vi "Initialize Attributes Core.vi"(8 "error in (no error)":errorcluster, 10 "Attribute Data":variant, 11 "BNT_ULx-MCSV in":refnum<class "BNT_ULx-MCSV.lvclass">) -> (0 "error out":errorcluster, 2 "MandatoryParameters":cluster{"Parameter":string, "found?":bool}[](array[cluster]), 3 "BNT_ULx-MCSV out":refnum<class "BNT_ULx-MCSV.lvclass">)   [LabVIEW 2021, in "BNT_ULx.lvlib" / "BNT_ULx-MCSV.lvclass"]
doc: "Initialize object attribute.\n\nUnique resources should be allocated elsewhere!"
uses:
  BNT_ULx-MCSV.lvclass
  C:/Users/Holger/Documents/LVP/CSPP/CSPP-Template/Packages/CSPP_Core/Actors/CSPP_DeviceActor/CSPP_DeviceActor.lvclass
  C:/Users/Holger/Documents/LVP/CSPP/CSPP-Template/Packages/CSPP_Core/Actors/CSPP_BaseActor/CSPP_BaseActor.lvclass
  CSPP_Core/Actors/CSPP_DeviceActor/CSPP_DeviceActor.lvclass/CSPP_DeviceActor.ctl
  CSPP_Core/Actors/CSPP_BaseActor/CSPP_BaseActor.lvclass/CSPP_BaseActor.ctl
  BNT_ULx-MCSV.lvclass/BNT_ULx-MCSV.ctl
  CSPP_Core/Libraries/Base/Severity.ctl
  CSPP_Core/Actors/CSPP_DeviceActor/CSPP_DeviceActor.lvclass
  CSPP_Core/Classes/CSPP_BaseClasses/Factory/CSPP_Factory.lvclass
  CSPP_Core/Actors/CSPP_BaseActor/CSPP_BaseActor.lvclass
  CSPP_Core/Libraries/Utilities/CSPP_Utilities.lvlib
  CSPP_Core/Libraries/Base/CSPP_Base.lvlib
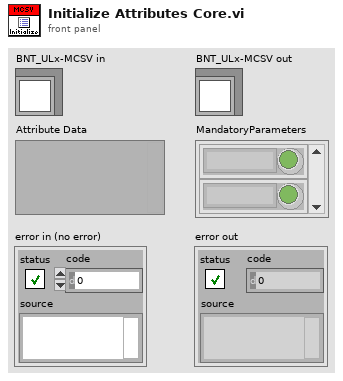
[diagram p1: front panel]
types:
  T1 = typedef "CSPP_Base.lvlib/Severity.ctl" = enum16{"emergency", "alert", "critical", "error", "warning", "notice", "info", "debug"}
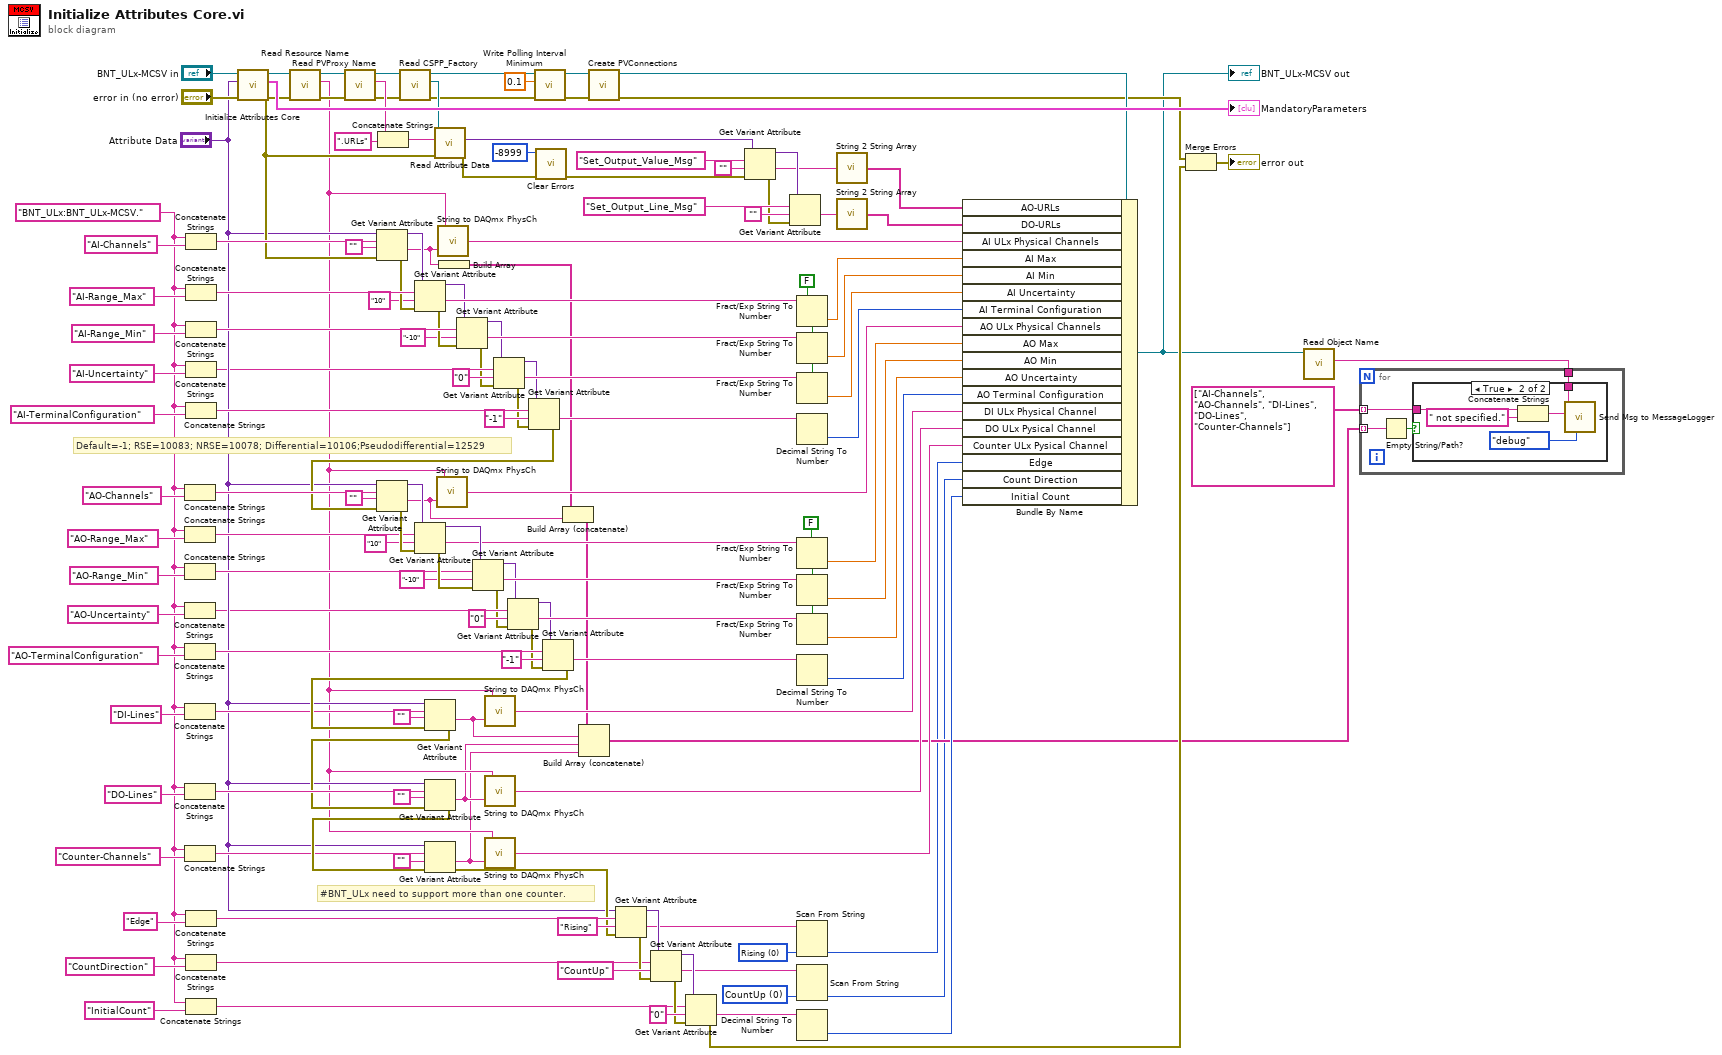
[diagram p0: block diagram]
diagram:
  w2 = 0 items=["CountUp", "CountDown"] ("Count Direction")
  w5 = 0 items=["Rising", "Falling"] ("Edge")
  w26 = FALSE ("use system decimal point (T)")
  w36 = FALSE ("use system decimal point (T)")
  w22 = "BNT_ULx:BNT_ULx-MCSV."
  # "#BNT_ULx need to support more than one counter."
  # "Default=-1; RSE=10083; NRSE=10078; Differential=10106;Pseudodifferential=12529"
  n1 = Concatenate Strings(w22, "AO-Channels" ("string")) -> (w130:string)
  n2 = Concatenate Strings(w22, "AO-Range_Max" ("string")) -> (w121:string)
  n3 = Concatenate Strings(w22, "AO-Range_Min" ("string")) -> (w124:string)
  n4 = Concatenate Strings(w22, "AO-Uncertainty" ("string")) -> (w28:string)
  n5 = Concatenate Strings(w22, "AO-TerminalConfiguration" ("string")) -> (w127:string)
  n6 = Concatenate Strings(w22, "DI-Lines" ("string")) -> (w108:string)
  n7 = Concatenate Strings(w22, "DO-Lines" ("string")) -> (w109:string)
  n8 = Concatenate Strings(w22, "Counter-Channels" ("string")) -> (w61:string)
  n9 = Concatenate Strings(w22, "AI-Channels" ("string")) -> (w138:string)
  n10 = Concatenate Strings(w22, "AI-Range_Max" ("string")) -> (w149:string)
  n11 = Concatenate Strings(w22, "AI-Range_Min" ("string")) -> (w146:string)
  n12 = Concatenate Strings(w22, "AI-Uncertainty" ("string")) -> (w38:string)
  n13 = Concatenate Strings(w22, "AI-TerminalConfiguration" ("string")) -> (w143:string)
  n14 = Concatenate Strings(w22, "Edge" ("string")) -> (w73:string)
  n15 = Concatenate Strings(w22, "CountDirection" ("string")) -> (w68:string)
  n16 = Concatenate Strings(w22, "InitialCount" ("string")) -> (w70:string)
  n17 = call-parent "Initialize Attributes Core.vi"("error in (no error)"="error in (no error)", "Attribute Data"="Attribute Data", "CSPP_DeviceActor in"="BNT_ULx-MCSV in") -> ("error out"=w54:errorcluster, "MandatoryParameters"=→"MandatoryParameters":cluster{"Parameter":string, "found?":bool}[], "CSPP_DeviceActor out"=w134:refnum<class "BNT_ULx-MCSV.lvclass">)  [unwired: 6 in]
  n18 = call "Read Resource Name.vi"("error in (no error)"=w54, "CSPP_DeviceActor in"=w134) -> ("error out"=w55:errorcluster, "Resource Name"=w18:string, "CSPP_DeviceActor out"=w106:refnum<class "BNT_ULx-MCSV.lvclass">)  [unwired: 7 in]
  n19 = call "Read PVProxy Name.vi"("error in (no error)"=w55, "CSPP_BaseActor in"=w106) -> ("error out"=w47:errorcluster, "PVProxy Name"=w101:string, "CSPP_BaseActor out"=w50:refnum<class "BNT_ULx-MCSV.lvclass">)  [unwired: 7 in]
  n20 = Get Variant Attribute(Variant="Attribute Data", name=w138, default value (empty Variant)="", error in=w54) -> (duplicate Variant=w137:variant, value=w14:string, error out=w136:errorcluster)  [unwired: 1 out]
  n21 = Concatenate Strings(w101, ".URLs" ("string")) -> (w103:string)
  n22 = call "Read CSPP_Factory.vi"("error in (no error)"=w47, "CSPP_BaseActor in"=w50) -> ("error out"=w46:errorcluster, "CSPP_Factory"=w48:refnum<class "CSPP_Factory.lvclass">, "CSPP_BaseActor out"=w49:refnum<class "BNT_ULx-MCSV.lvclass">)  [unwired: 7 in]
  n23 = Get Variant Attribute(Variant=w137, name=w149, default value (empty Variant)="10" ("string"), error in=w136) -> (duplicate Variant=w147:variant, value=w148:string, error out=w145:errorcluster)  [unwired: 1 out]
  n24 = call-dynamic "Read Attribute Data.vi"("error in (no error)"=w54, "Object Name"=w103, "CSPP_Factory in"=w48) -> ("error out"=w105:errorcluster, "Attribute Data"=w99:variant)  [unwired: 6 in, 1 out]
  n25 = call "String to DAQmx PhysCh.vi"("Channel String"=w14, "Resource Name"=w18) -> ("DAQmx Physical Channels"=w19:string)
  n26 = Build Array(w14) -> (w12:string[])
  n27 = Get Variant Attribute(Variant=w147, name=w146, default value (empty Variant)="-10" ("string"), error in=w145) -> (duplicate Variant=w33:variant, value=w144:string, error out=w32:errorcluster)  [unwired: 1 out]
  n28 = Get Variant Attribute(Variant=w33, name=w38, default value (empty Variant)="0" ("string"), error in=w32) -> (duplicate Variant=w35:variant, value=w39:string, error out=w34:errorcluster)  [unwired: 1 out]
  n29 = Get Variant Attribute(Variant=w35, name=w143, default value (empty Variant)="-1" ("string"), error in=w34) -> (value=w142:string, error out=w116:errorcluster)  [unwired: 2 out]
  n30 = Get Variant Attribute(Variant="Attribute Data", name=w130, default value (empty Variant)="", error in=w116) -> (duplicate Variant=w131:variant, value=w13:string, error out=w132:errorcluster)  [unwired: 1 out]
  n31 = Get Variant Attribute(Variant=w131, name=w121, default value (empty Variant)="10" ("string"), error in=w132) -> (duplicate Variant=w123:variant, value=w122:string, error out=w125:errorcluster)  [unwired: 1 out]
  n32 = call "String to DAQmx PhysCh.vi"("Channel String"=w13, "Resource Name"=w18) -> ("DAQmx Physical Channels"=w44:string)
  n33 = Get Variant Attribute(Variant=w123, name=w124, default value (empty Variant)="-10" ("string"), error in=w125) -> (duplicate Variant=w21:variant, value=w126:string, error out=w20:errorcluster)  [unwired: 1 out]
  n34 = Get Variant Attribute(Variant=w21, name=w28, default value (empty Variant)="0" ("string"), error in=w20) -> (duplicate Variant=w24:variant, value=w27:string, error out=w23:errorcluster)  [unwired: 1 out]
  n35 = call "Write Polling Interval Minimum.vi"("error in (no error)"=w46, "Polling Interval Minimum"=dbl[unit] 0.1, "CSPP_BaseActor in"=w49) -> ("error out"=w56:errorcluster, "CSPP_BaseActor out"=w58:refnum<class "BNT_ULx-MCSV.lvclass">)  [unwired: 7 in]
  n36 = call <vilib>:"Clear Errors.vi"("error in (no error)"=w105, "specific error code to clear (0: all)"=-8999) -> ("error out"=w98:errorcluster)  [unwired: 4 in, 1 out]
  n37 = Get Variant Attribute(Variant=w24, name=w127, default value (empty Variant)="-1" ("string"), error in=w23) -> (value=w128:string, error out=w113:errorcluster)  [unwired: 2 out]
  n38 = Get Variant Attribute(Variant="Attribute Data", name=w108, default value (empty Variant)="", error in=w113) -> (value=w10:string, error out=w107:errorcluster)  [unwired: 2 out]
  n39 = Get Variant Attribute(Variant="Attribute Data", name=w109, default value (empty Variant)="", error in=w107) -> (value=w9:string, error out=w63:errorcluster)  [unwired: 2 out]
  n40 = Get Variant Attribute(Variant="Attribute Data", name=w61, default value (empty Variant)="", error in=w63) -> (value=w8:string, error out=w64:errorcluster)  [unwired: 2 out]
  n41 = call "String to DAQmx PhysCh.vi"("Channel String"=w10, "Resource Name"=w18) -> ("DAQmx Physical Channels"=w43:string)
  n42 = call "String to DAQmx PhysCh.vi"("Channel String"=w9, "Resource Name"=w18) -> ("DAQmx Physical Channels"=w42:string)
  n43 = call "String to DAQmx PhysCh.vi"("Channel String"=w8, "Resource Name"=w18) -> ("DAQmx Physical Channels"=w41:string)
  n44 = Build Array (concatenate)(w12, w13) -> (w11:string[])
  n45 = Build Array (concatenate)(w11, w10, w9, w8) -> (w7:string[])
  n46 = call "Create PVConnections.vi"("error in (no error)"=w56, "BNT_ULx-MCSV in"=w58) -> ("error out"=w53:errorcluster, "BNT_ULx-MCSV out"=w57:refnum<class "BNT_ULx-MCSV.lvclass">)  [unwired: 8 in]
  n47 = Get Variant Attribute(Variant="Attribute Data", name=w73, default value (empty Variant)="Rising", error in=w64) -> (duplicate Variant=w62:variant, value=w6:string, error out=w74:errorcluster)  [unwired: 1 out]
  n48 = Get Variant Attribute(Variant=w62, name=w68, default value (empty Variant)="CountUp", error in=w74) -> (duplicate Variant=w69:variant, value=w3:string, error out=w71:errorcluster)  [unwired: 1 out]
  n49 = Get Variant Attribute(Variant=w69, name=w70, default value (empty Variant)="0", error in=w71) -> (value=w77:string, error out=w52:errorcluster)  [unwired: 2 out]
  n50 = Get Variant Attribute(Variant=w99, name="Set_Output_Value_Msg", default value (empty Variant)="", error in=w98) -> (duplicate Variant=w94:variant, value=w92:string, error out=w93:errorcluster)  [unwired: 1 out]
  n51 = Get Variant Attribute(Variant=w94, name="Set_Output_Line_Msg", default value (empty Variant)="", error in=w93) -> (value=w91:string)  [unwired: 3 out]
  n52 = Fract/Exp String To Number(use system decimal point (T)=w36, string=w148) -> (number=w88:dbl)  [unwired: 2 in, 1 out]
  n53 = Fract/Exp String To Number(use system decimal point (T)=w36, string=w144) -> (number=w87:dbl)  [unwired: 2 in, 1 out]
  n54 = Fract/Exp String To Number(use system decimal point (T)=w36, string=w39) -> (number=w31:dbl)  [unwired: 2 in, 1 out]
  n55 = Decimal String To Number(string=w142) -> (number=w141:i32)  [unwired: 2 in, 1 out]
  n56 = Fract/Exp String To Number(use system decimal point (T)=w26, string=w122) -> (number=w86:dbl)  [unwired: 2 in, 1 out]
  n57 = Fract/Exp String To Number(use system decimal point (T)=w26, string=w126) -> (number=w85:dbl)  [unwired: 2 in, 1 out]
  n58 = Fract/Exp String To Number(use system decimal point (T)=w26, string=w27) -> (number=w25:dbl)  [unwired: 2 in, 1 out]
  n59 = Decimal String To Number(string=w128) -> (number=w117:i32)  [unwired: 2 in, 1 out]
  n60 = Scan From String(input string=w6, default 1=w5) -> (output 1=w4:i32)  [unwired: 3 in, 3 out]
  n61 = Scan From String(input string=w3, default 1=w2) -> (output 1=w1:i32)  [unwired: 3 in, 3 out]
  n62 = Decimal String To Number(string=w77) -> (number=w59:i32)  [unwired: 2 in, 1 out]
  n63 = call "String 2 String Array.vi"("String"=w92) -> ("Substrings"=w90:string[])  [unwired: 1 in]
  n64 = call "String 2 String Array.vi"("String"=w91) -> ("Substrings"=w89:string[])  [unwired: 1 in]
  n65 = Bundle By Name(cluster=w57, "AO-URLs"=w90, "DO-URLs"=w89, "AI ULx Physical Channels"=w19, "AI Max"=w88, "AI Min"=w87, "AI Uncertainty"=w31, "AI Terminal Configuration"=w141, "AO ULx Physical Channels"=w44, "AO Max"=w86, "AO Min"=w85, "AO Uncertainty"=w25, "AO Terminal Configuration"=w117, "DI ULx Physical Channel"=w43, "DO ULx Pysical Channel"=w42, "Counter ULx Pysical Channel"=w41, "Edge"=w4, "Count Direction"=w1, "Initial Count"=w59) -> (w17:refnum<class "BNT_ULx-MCSV.lvclass">)
  "BNT_ULx-MCSV out" <- w17
  n66 = Merge Errors(w53, w52) -> (→"error out":errorcluster)
  n67 = call "Read Object Name.vi"("CSPP_BaseActor in"=w17) -> ("Object Name"=w16:string)  [unwired: 8 in, 2 out]
  n68 = for {
    tunnel: w16 -> [w158]
    tunnel: string[] ["AI-Channels", "AO-Channels", "DI-Lines", "DO-Lines", "Counter-Channels"] -> [w156] mode=indexing
    tunnel: w7 -> [w155] mode=indexing
    n69 = Empty String/Path?(string/path=w155) -> (empty?=w157:bool)
    n70 = case shown="True" w157 {
      tunnel: w158 -> [_ w163]
      tunnel: w156 -> [_ w162]
      frame False {
      }
      frame True {
        n71 = Concatenate Strings(w162, " not specified." ("string")) -> (w160:string)
        n72 = call "Send Msg to MessageLogger.vi"("Severity Code (info)"=Severity."debug", "Message Content"=w160, "Message Tag"=w163) -> ()  [unwired: 8 in, 1 out]
      }
    }
  }
